vi "homework - wf chart with running average.vi"() -> ()   [LabVIEW 2024]
doc: "#vi_description \nPlot a random number onto a waveform chart. Perform a running average of the most recent 4 points of data.\nThetic Engineering Ltd."
panel:
  in  "Stop":bool
  out "alarm":bool
  in  "threshold":dbl(knob)=0.49568843009143065 min=0.1 step=0.1 scale=0.1..0.9
  out "Waveform Chart":T1(graph)
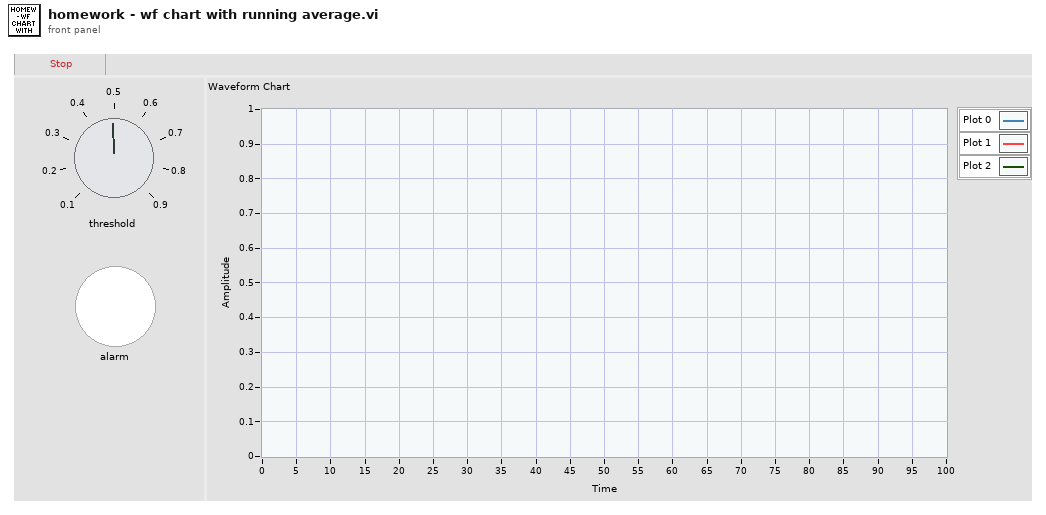
[diagram p1: front panel]
types:
  T1 = cluster{"number: 0 to 1":dbl, "threshold":dbl, dbl}
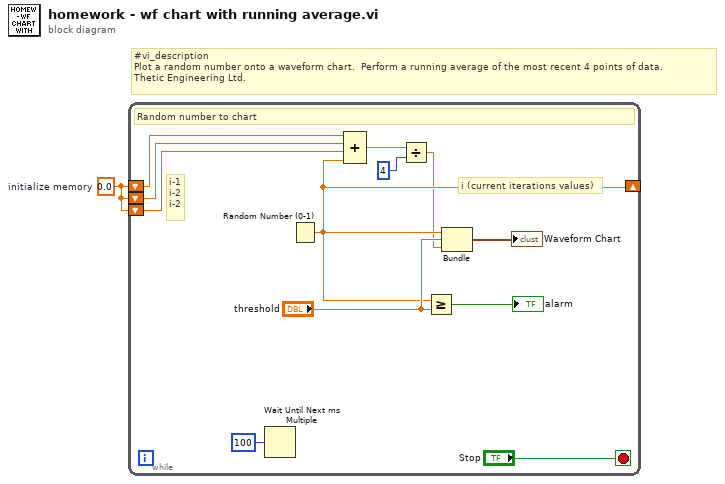
[diagram p0: block diagram]
diagram:
  w1 = 0.0  # initialize memory
  # "#vi_description \nPlot a random number onto a waveform chart.  Perform a running average of the most recent 4 points of data.\nThetic Engineering Ltd."
  n1 = while {
    shift-right: [w8] -> _
    shift-left: w1 -> [w5]
    shift-left: w1 -> [w6]
    shift-left: w1 -> [w7]
    stop <- "Stop" stop-if-true
    # "i (current iterations values)"
    # "i-1\ni-2\ni-2"
    # "Random number to chart"
    n2 = Wait Until Next ms Multiple(millisecond multiple=u32 100) -> ()  [unwired: 1 out]
    n3 = Random Number (0-1)() -> (number: 0 to 1=w8:dbl)
    n4 = Compound Arithmetic op=ADD(w5, w6, w7, w8) -> (w4:dbl)
    n5 = Divide(x=w4, y=4) -> (x/y=w3:dbl)
    n6 = Greater Or Equal?(x=w8, y="threshold") -> (x >= y?=→"alarm":bool)
    n7 = Bundle("number: 0 to 1"=w8, "threshold"="threshold", w3) -> (→"Waveform Chart":T1)  [unwired: 1 in]
  }
